vi "CheckHierarchyStatus.vi"() -> ()   [LabVIEW 2022 SP3]
uses:
  Anemometry Sub Vis/Globals/Constants_global.vi
  <vilib>/Utility/file.llb/Read Delimited Spreadsheet (string).vi
panel:
  in  "Resave if changed":bool=TRUE
  in  "recommenceAfter":path
  in  "Disable Automatic Error Handling":bool=TRUE
  in  "Remove Compiled Code":bool=TRUE
  in  "done":bool
  in  "start":bool
  in  "Mode":string(combo)="Recheck Good only"
  in  "save:":bool
  out "Broken VIs found":i32
  out "healthcheckSavingTo":path
  out "nFilesChecked":i32
  in  "healthcheckThis:":path=path "" caption="healthcheck or re-check This:"
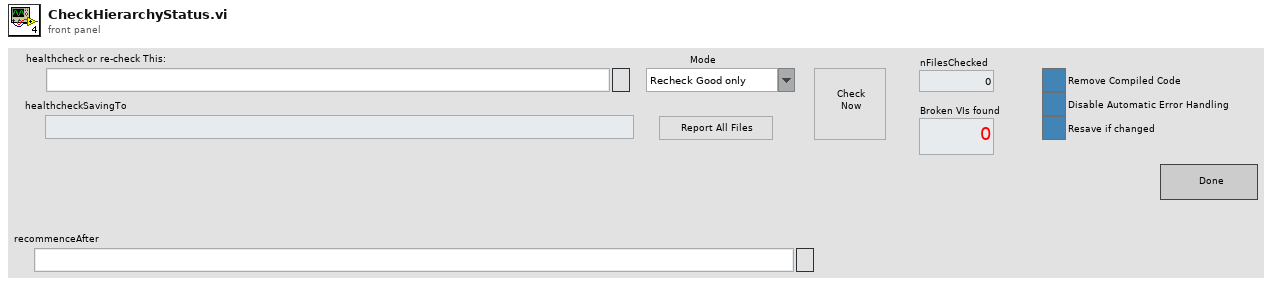
[diagram p1: front panel]
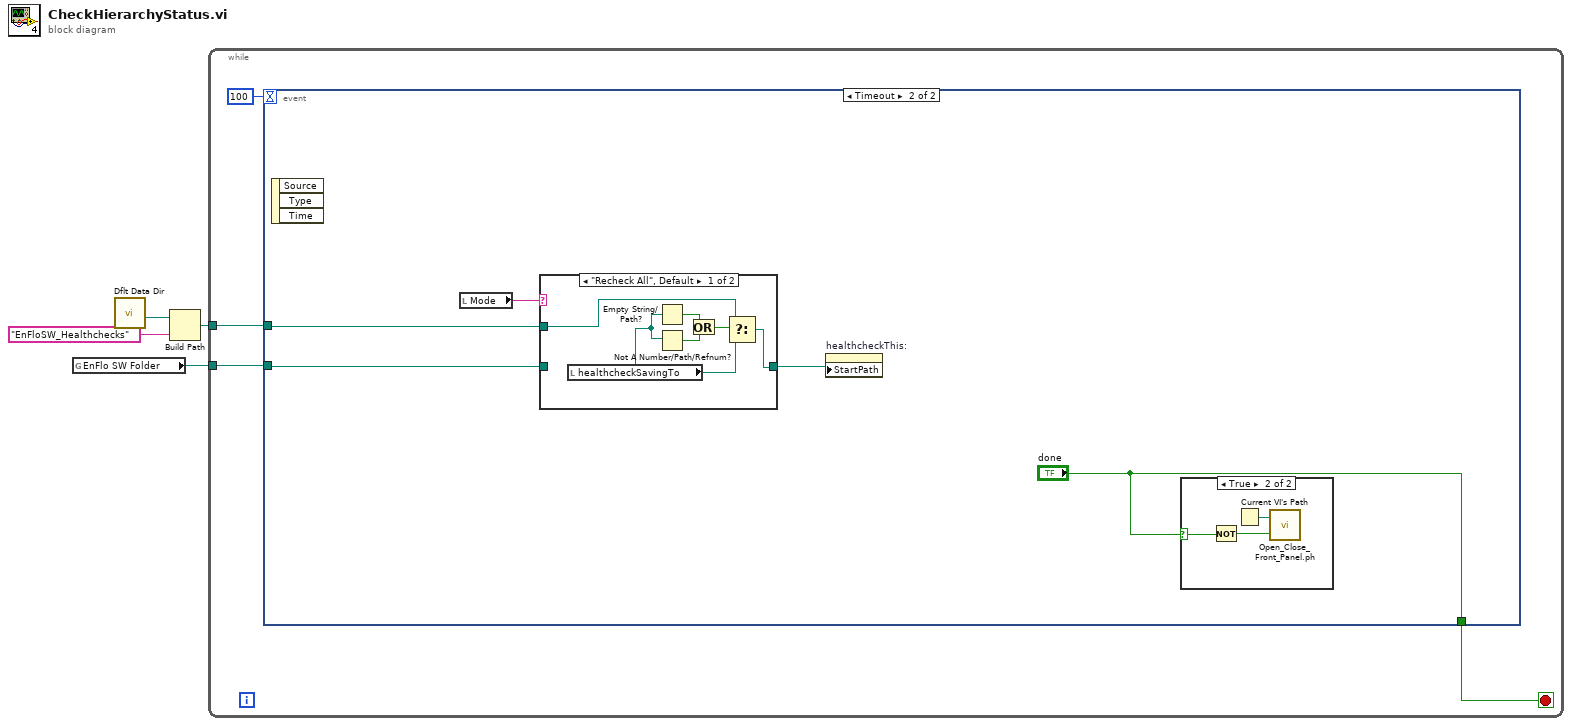
[diagram p0: block diagram]
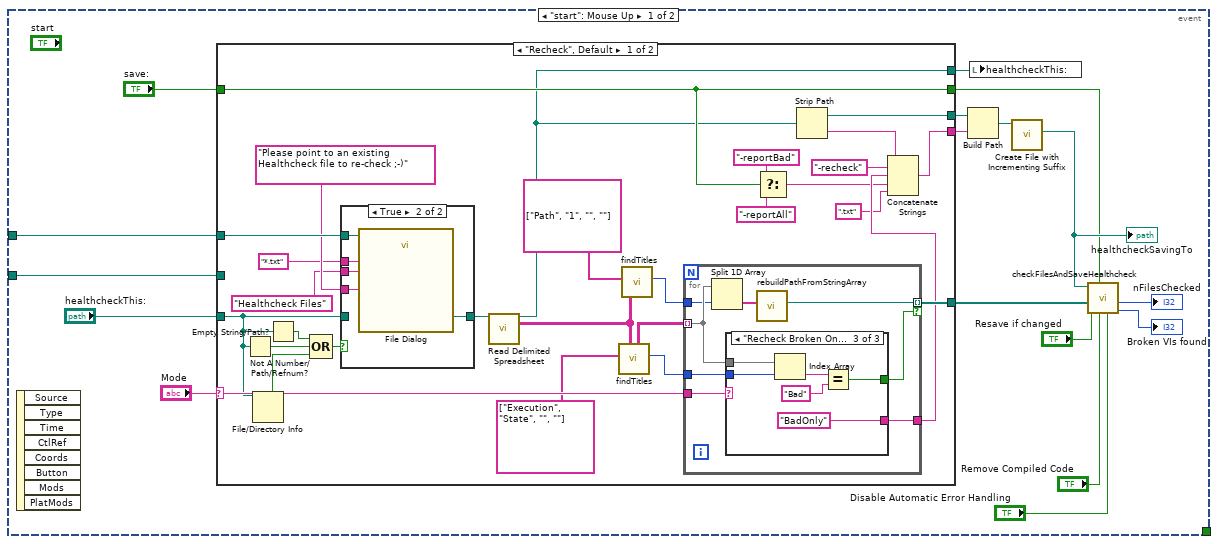
[diagram p2: hidden frame]
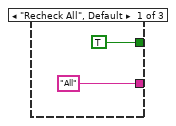
[diagram p4: hidden frame]
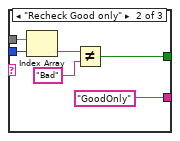
[diagram p5: hidden frame]
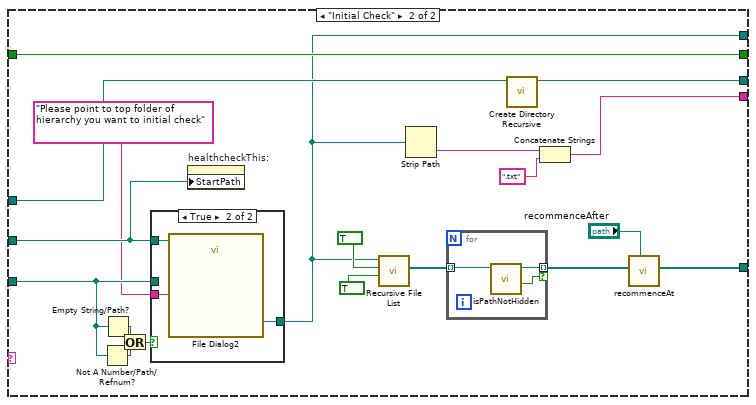
[diagram p6: hidden frame]
diagram:
  n1 = global read "Constants_global.vi" "EnFlo SW Folder"() -> (w1:path)
  n2 = call <vilib>:"Dflt Data Dir.vi"() -> ("App:Default Data Directory"=w4:path)
  n3 = Build Path(base path=w4, name or relative path="EnFloSW_Healthchecks") -> (appended path=w2:path)
  n4 = while {
    tunnel: w2 -> [w6]
    tunnel: w1 -> [w5]
    stop <- w7 stop-if-true
    n5 = event shown="[1] Timeout" {
      selector: _ -> [_ _]
      dyn-events: _ -> [_ _]
      timeout: 100 -> [_ _]
      tunnel: [_ "done"] -> w7
      tunnel: w6 -> [w13 w110]
      tunnel: w5 -> [w12 w111]
      event "start": Mouse Up {
        n6 = event-data() -> ()  [unwired: 1 in, 8 out]
        n7 = case shown="\"Recheck\", Default" "Mode" {
          selector: "Mode" -> [w47 _]
          tunnel: [w51 w99] -> w24
          tunnel: "healthcheckThis:" -> [w27 w91]
          tunnel: [w49 w85] -> w21
          tunnel: [w52 w97] -> w18
          tunnel: [w50 w95] -> w17
          tunnel: "save:" -> [w50 w95]
          tunnel: [w48 w92] -> w15
          tunnel: w13 -> [w44 w94]
          tunnel: w12 -> [_ w88]
          frame "Recheck", Default {
            n8 = Not A Number/Path/Refnum?(number/path/refnum=w27) -> (NaN/Path/Refnum?=w26:bool)
            n9 = File/Directory Info(path=w27) -> (directory=w31:bool)  [unwired: 1 in, 6 out]
            n10 = Empty String/Path?(string/path=w27) -> (empty?=w46:bool)
            n11 = Compound Arithmetic op=OR(w46, w26, w31) -> (w32:bool)
            n12 = case shown="True" w32 {
              tunnel: w44 -> [_ w60]
              tunnel: [w55 w59] -> w45
              tunnel: w27 -> [w55 _]
              tunnel: "Please point to an existing Healthcheck file to re-check ;-)" ("prompt") -> [_ w58]
              tunnel: "*.txt" ("pattern (all files)") -> [_ w57]
              tunnel: "Healthcheck Files" ("pattern label") -> [_ w56]
              frame False {
              }
              frame True {
                n13 = call "File Dialog"("start path"=w60, "prompt"=w58, "pattern (all files)"=w57, "pattern label"=w56) -> ("selected path"=w59:path)  [unwired: 8 in, 3 out]
              }
            }
            n14 = call-poly <vilib>:"Read Delimited Spreadsheet.vi"("file path (dialog if empty)"=w45) -> ("new file path (Not A Path if cancelled)"=w48:path, "all rows"=w40:string[][])  [unwired: 9 in, 4 out]
            n15 = call "findTitles.vi"("all rows in"=w40, "Array - String"=string[] ["Execution", "State", "", ""]) -> ("titleColumn"=w42:i32, "data"=w38:string[][])  [unwired: 8 in]
            n16 = call "findTitles.vi"("all rows in"=w40, "Array - String"=string[] ["Path", "1", "", ""]) -> ("titleColumn"=w41:i32)  [unwired: 8 in, 1 out]
            n17 = for {
              tunnel: w38 -> [w67] mode=indexing
              tunnel: [w68] -> w49 mode=indexing if=w64
              tunnel: w41 -> [w66]
              tunnel: w42 -> [w65]
              tunnel: w47 -> [w62]
              tunnel: [w61] -> w35
              n18 = Split 1D Array(array=w67, index=w66) -> (second subarray=w63:string[])  [unwired: 1 out]
              n19 = case shown="\"Recheck Broken Only\"" w62 {
                tunnel: w67 -> [_ w76 w82]
                tunnel: w65 -> [_ w73 w79]
                tunnel: [TRUE w72 w78] -> w64
                tunnel: ["All" ("y") "GoodOnly" ("y") "BadOnly" ("y")] -> w61
                frame "Recheck All", Default {
                }
                frame "Recheck Good only" {
                  n20 = Index Array(array=w76, index=w73) -> (element=w75:string)
                  n21 = Not Equal?(x=w75, y="Bad") -> (x != y?=w72:bool)
                }
                frame "Recheck Broken Only" {
                  n22 = Index Array(array=w82, index=w79) -> (element=w81:string)
                  n23 = Equal?(x=w81, y="Bad") -> (x = y?=w78:bool)
                }
              }
              n24 = call "rebuildPathFromStringArray.vi"("stringArray"=w63) -> ("path"=w68:path)  [unwired: 10 in]
            }
            n25 = Select(t="-reportBad" ("string"), s=w50, f="-reportAll" ("string")) -> (s? t:f=w33:string)
            n26 = Strip Path(path=w48) -> (stripped path=w52:path, name=w37:string)
            n27 = Concatenate Strings(w37, "-recheck" ("string"), w35, w33, ".txt" ("string")) -> (w51:string)
          }
          frame "Initial Check" {
            n28 = Not A Number/Path/Refnum?(number/path/refnum=w91) -> (NaN/Path/Refnum?=w89:bool)
            n29 = Empty String/Path?(string/path=w91) -> (empty?=w93:bool)
            n30 = Or(x=w93, y=w89) -> (x .or. y?=w90:bool)
            n31 = case shown="True" w90 {
              tunnel: w88 -> [_ w108]
              tunnel: [w105 w107] -> w92
              tunnel: w91 -> [w105 _]
              tunnel: "Please point to top folder of hierarchy you want to initial check" ("prompt") -> [_ w106]
              frame False {
              }
              frame True {
                n32 = call "File Dialog2"("start path"=w108, "prompt"=w106) -> ("selected path"=w107:path)  [unwired: 10 in, 3 out]
              }
            }
            n33 = property on="healthcheckThis:" class="Path"("StartPath"=w88) -> ()  [unwired: 2 in, 2 out]
            n34 = call <vilib>:"Recursive File List.vi"("Continue Recursing on Error? (F)"=TRUE, "Treat LLBs as Folders?"=TRUE, "Folder Path"=w92) -> ("All Files in Dir"=w86:path[])  [unwired: 4 in, 4 out]
            n35 = Strip Path(path=w92) -> (name=w96:string)  [unwired: 1 out]
            n36 = for {
              tunnel: w86 -> [w104] mode=indexing
              tunnel: [w103] -> w84 mode=indexing if=w102
              n37 = call "isPathNotHidden.vi"("pathIn"=w104) -> ("pathNotHidden"=w102:bool, "pathOut"=w103:path)  [unwired: 8 in, 1 out]
            }
            n38 = call <vilib>:"Create Directory Recursive.vi"("directory"=w94) -> ("directory copy"=w97:path)  [unwired: 4 in, 2 out]
            n39 = Concatenate Strings(w96, ".txt" ("string")) -> (w99:string)
            n40 = call "recommenceAt.vi"("splitAtFile"="recommenceAfter", "Array"=w84) -> ("Array 2"=w85:path[])  [unwired: 9 in]
          }
        }
        n41 = Build Path(base path=w18, name or relative path=w24) -> (appended path=w25:path)
        n42 = local write "healthcheckThis:"(w15) -> ()
        n43 = call <vilib>:"Create File with Incrementing Suffix.vi"("file path"=w25) -> ("actual path"=w23:path)  [unwired: 8 in, 2 out]
        "healthcheckSavingTo" <- w23
        n44 = call "checkFilesAndSaveHealthcheck.vi"("Disable Automatic Error Handling"="Disable Automatic Error Handling", "Remove Compiled Code"="Remove Compiled Code", "saveBadOnly?"=w17, "Resave if changed"="Resave if changed", "filesToCheck"=w21, "saveTo"=w23) -> ("Broken VIs found"=→"Broken VIs found":i32, "Progress Bar"=→"nFilesChecked":i32)  [unwired: 3 in, 1 out]
      }
      event Timeout {
        n45 = event-data() -> ()  [unwired: 1 in, 3 out]
        n46 = local read "Mode"() -> (w113:string)
        n47 = case shown="\"Recheck All\", Default" w113 {
          tunnel: [w117 w123] -> w112
          tunnel: w111 -> [_ w123]
          tunnel: w110 -> [w118 _]
          frame "Recheck All", Default {
            n48 = local read "healthcheckSavingTo"() -> (w119:path)
            n49 = Empty String/Path?(string/path=w119) -> (empty?=w120:bool)
            n50 = Not A Number/Path/Refnum?(number/path/refnum=w119) -> (NaN/Path/Refnum?=w121:bool)
            n51 = Or(x=w120, y=w121) -> (x .or. y?=w122:bool)
            n52 = Select(t=w118, s=w122, f=w119) -> (s? t:f=w117:path)
          }
          frame "Initial Check" {
          }
        }
        n53 = property on="healthcheckThis:" class="Path"("StartPath"=w112) -> ()  [unwired: 2 in, 2 out]
        n54 = case shown="True" "done" {
          selector: "done" -> [_ w114]
          frame False {
          }
          frame True {
            n55 = Not(x=w114) -> (.not. x?=w116:bool)
            n56 = Current VI's Path() -> (path=w115:path)
            n57 = call "Open_Close_Front_Panel.ph.vi"("openWindow (T)"=w116, "VI path"=w115) -> ()  [unwired: 1 in, 1 out]
          }
        }
      }
    }
  }
